vi "FTW-Regex-Execute.vi"(0 "Regex":refnum<class "FTW-Regex.lvclass">, 5 "Subject String":string, 7 "Starting Offset":i32, 11 "error in":errorcluster) -> (4 "Regex out":refnum<class "FTW-Regex.lvclass">, 6 "Whole Match Begin":i32, 8 "Offset after Match":i32, 10 "Submatches":i32[](array[numeric]), 14 "Callouts":T1(array[cluster]), 15 "error out":errorcluster)   [LabVIEW 2014, in "FTW-Regex.lvclass"]
uses:
  FTW-Regex.lvclass
  FTW-Regex.lvclass/FTW-Regex.ctl
  error/FTW-ERR-ThrowError.vi
  error/FTW-ERR-NoErrorConstant.vi
  error/FTW-ERR-CallChain.vi
  string/FTW-STR-ReplaceWhitespace.vi
panel:
  # "Inputs"
  # "Outputs"
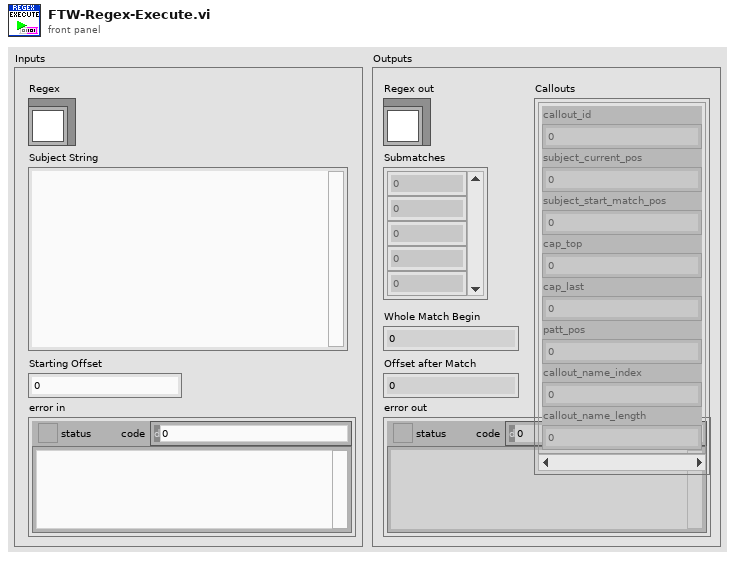
[diagram p1: front panel]
types:
  T1 = cluster{"callout_id":i32, "subject_current_pos":i32, "subject_start_match_pos":i32, "cap_top":i32, "cap_last":i32, "patt_pos":i32, "callout_name_index":i32, "callout_name_length":i32}[]
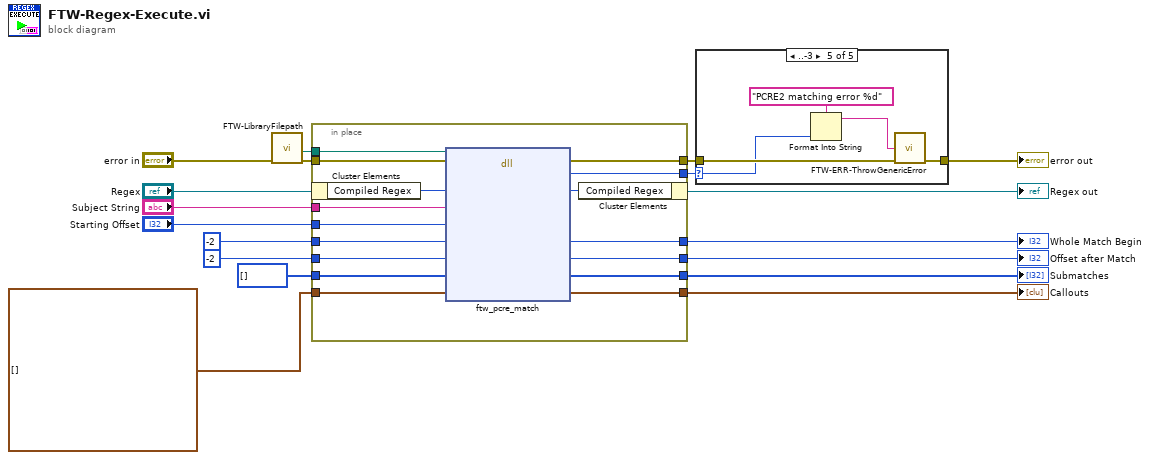
[diagram p0: block diagram]
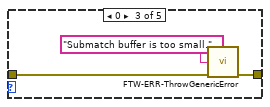
[diagram p4: hidden frame]
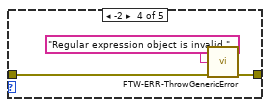
[diagram p5: hidden frame]
diagram:
  n1 = call "FTW-LibraryFilepath.vi"("error in"="error in") -> ("error out"=w16:errorcluster, "Library Filepath"=w17:path)  [unwired: 8 in, 1 out]
  n2 = in-place {
    in-place-border: [w34] -> w7
    in-place-border: w17 -> [w33]
    in-place-border: w16 -> [w32]
    in-place-border: "Subject String" -> [w29]
    in-place-border: "Starting Offset" -> [w28]
    in-place-border: [w26] -> w11
    in-place-border: i32[] [] -> [w27]
    in-place-border: [w25] -> w10
    in-place-border: [w24] -> w1
    in-place-border: [w23] -> w9
    in-place-border: [w22] -> w6
    in-place-border: -2 -> [w21]
    in-place-border: -2 -> [w20]
    in-place-border: T1 [] ("Callouts") -> [w19]
    n3 = in-place-cluster #1("Regex") -> ("Compiled Regex"=w31:u64)
    n4 = dll-call lib="?" fn="ftw_pcre_match"(path in=w33, error in=w32, "Compiled Regex"=w31, "Subject String"=w29, "Starting Offset"=w28, "Match Begin"=w21, "Match End"=w20, "Submatch Buffer"=w27, "Callout Buffer"=w19) -> (error out=w34:errorcluster, "Return Value"=w23:i32, "Compiled Regex"=w30:u64, "Match Begin"=w22:i32, "Match End"=w26:i32, "Submatch Buffer"=w25:i32[], "Callout Buffer"=w24:T1)  [unwired: 3 in, 1 out]
    n5 = in-place-cluster #1("Compiled Regex"=w30) -> (→"Regex out":refnum<class "FTW-Regex.lvclass">)
  }
  "Offset after Match" <- w11
  "Submatches" <- w10
  "Callouts" <- w1
  "Whole Match Begin" <- w6
  n6 = case shown="..-3" w9 {
    selector: w9 -> [_ _ _ _ w45]
    tunnel: [w35 w36 w38 w41 w46] -> w8
    tunnel: w7 -> [w35 w36 w39 w42 w47]
    frame 1.. {
      # "Match found and no error."
    }
    frame -1 {
      # "PCRE_ERROR_NOMATCH\nDon't treat this as an error!"
    }
    frame 0 {
      n7 = call "FTW-ERR-ThrowGenericError.vi"("Error Message"="Submatch buffer is too small.", "error in"=w39) -> ("error out"=w38:errorcluster)  [unwired: 13 in]
    }
    frame -2 {
      n8 = call "FTW-ERR-ThrowGenericError.vi"("Error Message"="Regular expression object is invalid.", "error in"=w42) -> ("error out"=w41:errorcluster)  [unwired: 13 in]
    }
    frame ..-3 {
      n9 = Format Into String(format string="PCRE2 matching error %d" ("Error Message"), w45) -> (resulting string=w44:string)  [unwired: 2 in, 1 out]
      n10 = call "FTW-ERR-ThrowGenericError.vi"("Error Message"=w44, "error in"=w47) -> ("error out"=w46:errorcluster)  [unwired: 13 in]
    }
  }
  "error out" <- w8
